vi "Draw.vi"(7 "Stimulus Snippet":T1, 8 "error in (no error)":errorcluster, 9 "StimulusImageIn":T2, 10 "CalibrationImage":T2, 11 "DetectSuppressionDuration in":refnum<class "DetectSuppressionDuration.lvclass">) -> (0 "error out":errorcluster, 1 "StimulusImageOut":T2, 3 "DetectSuppressionDuration out":refnum<class "DetectSuppressionDuration.lvclass">)   [LabVIEW 2019, in "DetectSuppressionDuration.lvclass"]
uses:
  DetectSuppressionDuration.lvclass
  <vilib>/vision/Image Controls.llb/IMAQ Image.ctl
  StimulusSnippetCluster.ctl
  DetectSuppressionDuration.lvclass/DetectSuppressionDuration.ctl
  ParametersGlobal.vi
  <vilib>/vision/NI_Vision_Development_Module.lvlib
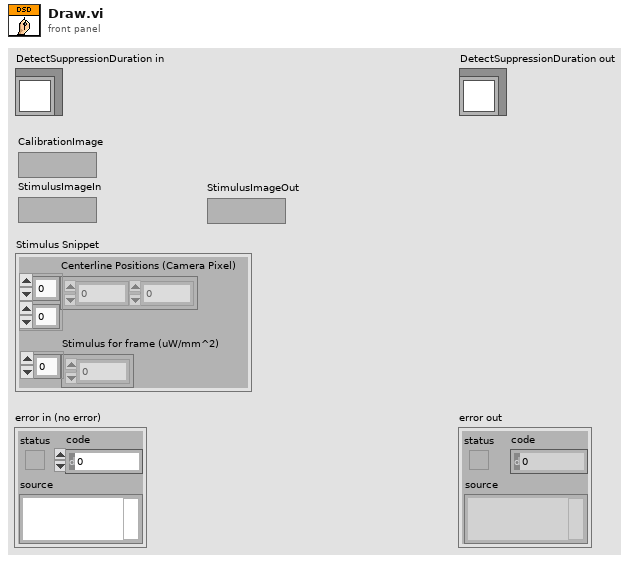
[diagram p1: front panel]
types:
  T1 = typedef "StimulusSnippetCluster.ctl" = cluster{"Centerline Positions (Camera Pixel)":sgl[][], "Stimulus for frame (uW/mm^2)":sgl[]}
  T2 = typedef "IMAQ Image.ctl" = refnum<image>
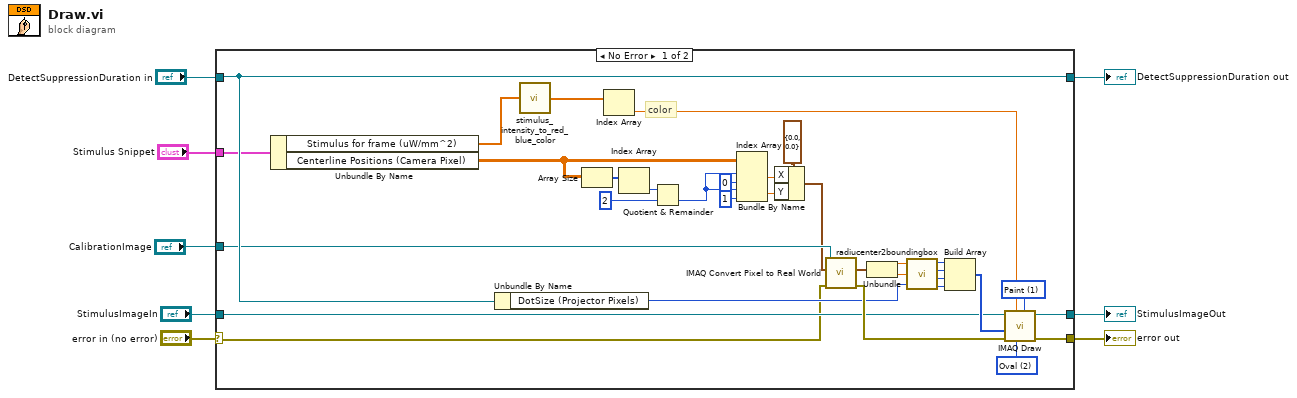
[diagram p0: block diagram]
diagram:
  n1 = case shown="No Error" "error in (no error)" {
    selector: "error in (no error)" -> [w22 w44]
    tunnel: [w10 w44] -> w2
    tunnel: [w23 w43] -> w3
    tunnel: "DetectSuppressionDuration in" -> [w23 w43]
    tunnel: [w11 w42] -> w1
    tunnel: "StimulusImageIn" -> [w29 w42]
    tunnel: "Stimulus Snippet" -> [w20 _]
    tunnel: "CalibrationImage" -> [w19 _]
    frame No Error {
      w9 = u16 1 items=["Frame", "Paint", "Invert Frame", "Invert Paint"] ("Draw Mode")
      w41 = u16 2 items=["Line", "Rectangle", "Oval"] ("Shape to draw")
      # "color"
      n2 = Unbundle By Name(w20) -> ("Stimulus for frame (uW/mm^2)"=w21:sgl[], "Centerline Positions (Camera Pixel)"=w16:sgl[][])
      n3 = Unbundle By Name(w23) -> ("DotSize (Projector Pixels)"=w24:i32)
      n4 = call "stimulus_intensity_to_red_blue_color.vi"("StimulusIntensityForFrame"=w21) -> ("StimulusColorForFrame"=w25:sgl[])
      n5 = Array Size(array=w16) -> (size(s)=w15:i32[])
      n6 = Index Array(array=w25) -> (element=w18:sgl)  [unwired: 1 in]
      n7 = Index Array(array=w15) -> (element=w14:i32)  [unwired: 1 in]
      n8 = Quotient & Remainder(x=w14, y=2) -> (floor(x/y)=w12:i32)  [unwired: 1 out]
      n9 = Index Array(array=w16, index (row) #1=w12, index (col) #1=0 ("disabled index (col)"), index (row) #2=w12, index (col) #2=1 ("disabled index (col)")) -> (element #1=w27:sgl, element #2=w26:sgl)
      n10 = Bundle By Name(cluster=cluster{"X":sgl, "Y":sgl} {"X"=0.0, "Y"=0.0} ("Camera Point"), "X"=w27, "Y"=w26) -> (w17:cluster{"X":sgl, "Y":sgl})
      n11 = call "IMAQ Convert Pixel to Real World"("error in (no error)"=w22, "Pixel Coordinates"=w17, "Calibrated Image"=w19) -> ("error out"=w32:errorcluster, "Real World Coordinates"=w33:cluster{"X":sgl, "Y":sgl})  [unwired: 3 in, 4 out]
      n12 = Unbundle(w33) -> ("X"=w35:sgl, "Y"=w34:sgl)
      n13 = call "radiucenter2boundingbox.vi"("Radius"=w24, "ycenter"=w34, "xcenter"=w35) -> ("Bottom"=w36:i32, "Right"=w37:i32, "Top"=w38:i32, "Left"=w39:i32)  [unwired: 2 in]
      n14 = Build Array(w39, w38, w37, w36) -> (w40:i32[])
      n15 = call "IMAQ Draw"("Draw Mode"=w9, "Shape to draw"=w41, "Pixel Color"=w18, "error in (no error)"=w32, "Coordinates"=w40, "Image Src"=w29) -> ("error out"=w10:errorcluster, "Image Dst Out"=w11:T2)  [unwired: 4 in]
    }
    frame Error {
    }
  }
  "error out" <- w2
  "DetectSuppressionDuration out" <- w3
  "StimulusImageOut" <- w1
